vi "Stop.vi"(8 "error in":errorcluster, 11 "Actor in":refnum<class "Actor.lvclass">) -> (3 "Actor out":refnum<class "Actor.lvclass">)   [LabVIEW 2013, in "Actor Framework.lvlib" / "Actor.lvclass"]
doc: "(<B>Filename</B>: Actor Framework.lvlib:Actor.lvclass:Stop.vi)\n\nWrapper for Stop Core.vi. This VI is called by the Do method of the Stop Msg class."
uses:
  <vilib>/ActorFramework/Actor/Actor.lvclass
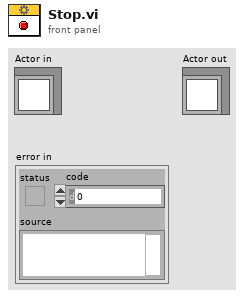
[diagram p1: front panel]
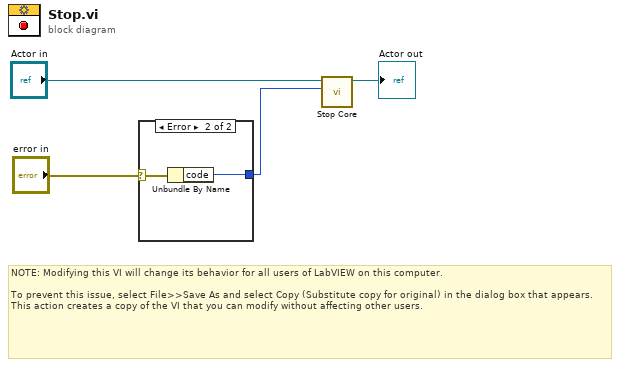
[diagram p0: block diagram]
diagram:
  # "NOTE: Modifying this VI will change its behavior for all users of LabVIEW on this computer.\n\nTo prevent this issue, select File>>Save As and select Copy (Substitute copy for original) in the dialog box that appears. This action creates a copy of the VI that you can modify without affecting other users."
  n1 = case shown="Error" "error in" {
    selector: "error in" -> [_ w6]
    tunnel: [_ w5] -> w1
    frame No Error {
    }
    frame Error {
      n2 = Unbundle By Name(w6) -> ("code"=w5:i32)
    }
  }
  n3 = call-dynamic "Stop Core.vi"("final error code"=w1, "Actor in"="Actor in") -> ("Actor out"=→"Actor out":refnum<class "Actor.lvclass">)  [unwired: 9 in]
